vi "Write Data Queue.vi"(8 "error in":errorcluster, 10 "Data Queue":refnum<queue>, 11 "Observer in":refnum<class "Observer.lvclass">) -> (0 "error out":errorcluster, 3 "Observer out":refnum<class "Observer.lvclass">)   [LabVIEW 2015, in "Observer.lvclass"]
uses:
  Observer.lvclass
  Data/Data.lvclass
  Observer.lvclass/Observer.ctl
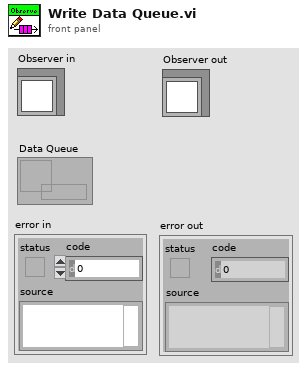
[diagram p1: front panel]
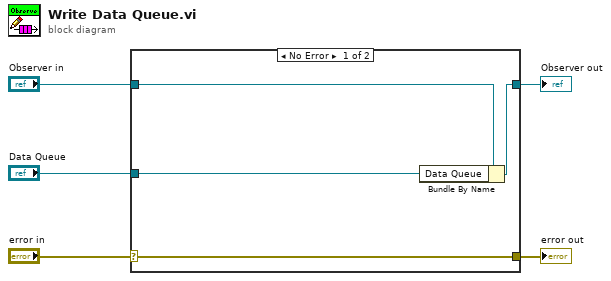
[diagram p0: block diagram]
diagram:
  n1 = case shown="No Error" "error in" {
    selector: "error in" -> [w9 w10]
    tunnel: [w9 w10] -> w4
    tunnel: [w7 w11] -> w2
    tunnel: "Observer in" -> [w8 w11]
    tunnel: "Data Queue" -> [w6 _]
    frame No Error {
      n2 = Bundle By Name(cluster=w8, "Data Queue"=w6) -> (w7:refnum<class "Observer.lvclass">)
    }
    frame Error {
    }
  }
  "error out" <- w4
  "Observer out" <- w2
